vi "NIMS_dfd_Convert Band Specs (Remez Weight).vi"(8 "s":string, 9 "Weight":dbl[](array[numeric]), 10 "A":dbl[](array[numeric]), 11 "F":dbl[](array[numeric])) -> (0 "error out":errorcluster, 1 "freqs of exact gain [Hz]":dbl[](array[numeric]), 2 "band specs":T1[](array[typedef])=[{"band specification"=[{"freq"=0.0, "amplitude"=1.0, "weight"=1.0}, {"freq"=0.2, "amplitude"=1.0, "weight"=1.0}], "ripple constraint"=0.0}, {"band specification"=[{"freq"=0.3, "amplitude"=0.0, "weight"=1.0}, {"freq"=0.5, "amplitude"=0.0, "weight"=1.0}], "ripple constraint"=0.0}])   [LabVIEW 2017, in "NI_DigFilter_MathScript.lvlib"]
uses:
  <vilib>/addons/Digital Filter Design/NI_DigFilter_MathScript.lvlib
  <vilib>/addons/Digital Filter Design/_Objects.llb/DFD Adv Band Spec.ctl
  <vilib>/addons/Digital Filter Design/_Misc.llb/dfd_Error Handlers (Multiple).vi
  <vilib>/addons/Digital Filter Design/NI_DigFilterLicensed.lvlib
panel:
  # "freq"
  # "amplitude"
  # "weight"
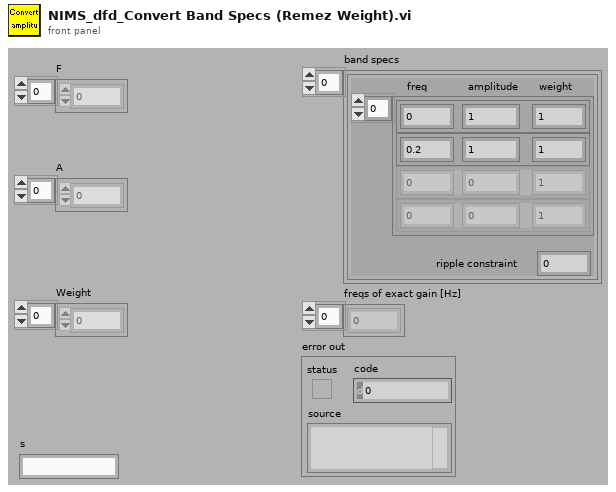
[diagram p1: front panel]
types:
  T1 = typedef "NI_DigFilterLicensed.lvlib/DFD Adv Band Spec.ctl" = cluster{"band specification":cluster{"freq":dbl, "amplitude":dbl, "weight":dbl}[], "ripple constraint":dbl}
  T2 = cluster{cluster{"Numeric":dbl, "Numeric":dbl, "f":dbl}[], dbl}[]
  T3 = cluster{cluster{"Numeric":dbl, "Numeric":dbl, "f":dbl}[], dbl}
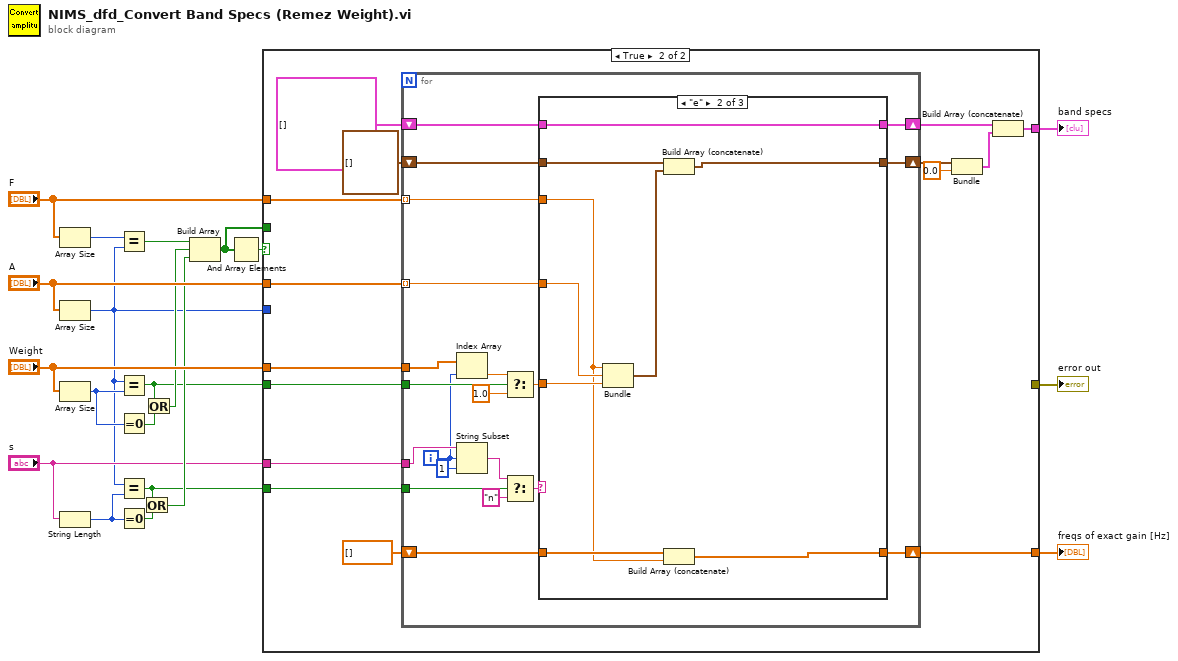
[diagram p0: block diagram]
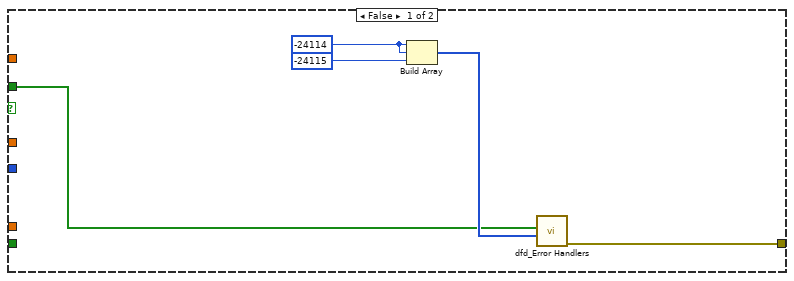
[diagram p2: hidden frame]
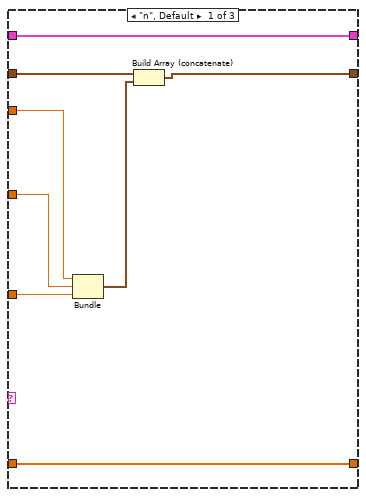
[diagram p3: hidden frame]
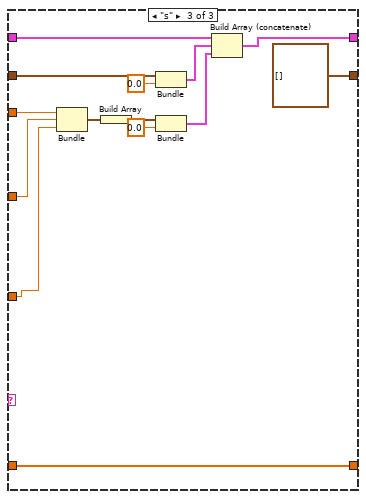
[diagram p4: hidden frame]
diagram:
  n1 = Array Size(array="F") -> (size(s)=w20:i32)
  n2 = Array Size(array="A") -> (size(s)=w6:i32)
  n3 = Array Size(array="Weight") -> (size(s)=w15:i32)
  n4 = String Length(string="s") -> (length=w14:i32)
  n5 = Equal?(x=w20, y=w6) -> (x = y?=w19:bool)
  n6 = Equal?(x=w6, y=w15) -> (x = y?=w8:bool)
  n7 = Equal To 0?(x=w15) -> (x = 0?=w9:bool)
  n8 = Equal?(x=w6, y=w14) -> (x = y?=w7:bool)
  n9 = Equal To 0?(x=w14) -> (x = 0?=w13:bool)
  n10 = Or(x=w7, y=w13) -> (x .or. y?=w11:bool)
  n11 = Or(x=w8, y=w9) -> (x .or. y?=w12:bool)
  n12 = Build Array(w19, w12, w11) -> (w1:bool[])
  n13 = And Array Elements(Boolean array=w1) -> (logical AND=w2:bool)
  n14 = case shown="True" w2 {
    tunnel: "F" -> [_ w40]
    tunnel: "A" -> [_ w39]
    tunnel: "Weight" -> [_ w38]
    tunnel: [w22 _] -> w16
    tunnel: "s" -> [_ w37]
    tunnel: w8 -> [_ w35]
    tunnel: w7 -> [_ w36]
    tunnel: w6 -> [_ _]
    tunnel: [_ w28] -> w4
    tunnel: [_ w27] -> w3
    tunnel: w1 -> [w21 _]
    frame False {
      w23 = -24114 ("element")
      n15 = Build Array(w23, w23, -24115 ("element")) -> (w25:i32[])
      n16 = call-poly <vilib>:"dfd_Error Handlers.vi"("error sources"=w25, "condition failed?"=w21) -> ("error out"=w22:errorcluster)  [unwired: 1 in, 8 out]
    }
    frame True {
      n17 = for {
        tunnel: w40 -> [w50] mode=indexing
        tunnel: w39 -> [w51] mode=indexing
        tunnel: w38 -> [w42]
        tunnel: w37 -> [w60]
        tunnel: w36 -> [w56]
        tunnel: w35 -> [w58]
        shift-right: [w48] -> w31
        shift-left: cluster{"Numeric":dbl, "Numeric":dbl, "f":dbl}[] [] -> [w49]
        shift-right: [w46] -> w27
        shift-left: dbl[] [] -> [w47]
        shift-right: [w44] -> w30
        shift-left: T2 [] -> [w45]
        i -> [w41]
        n18 = Index Array(array=w42, index=w41) -> (element=w43:dbl)
        n19 = String Subset(string=w60, offset (0)=w41, length (rest)=1 ("length (rest)")) -> (substring=w55:string)
        n20 = Select(t=w43, s=w58, f=1.0) -> (s? t:f=w52:dbl)
        n21 = Select(t=w55, s=w56, f="n") -> (s? t:f=w53:string)
        n22 = case shown="\"e\"" w53 {
          tunnel: w52 -> [w66 w76 w87]
          tunnel: w51 -> [w67 w77 w88]
          tunnel: w50 -> [w68 w70 w89]
          tunnel: w49 -> [w65 w75 w91]
          tunnel: [w63 w73 cluster{"Numeric":dbl, "Numeric":dbl, "f":dbl}[] []] -> w48
          tunnel: w47 -> [w62 w72 w78]
          tunnel: [w62 w71 w78] -> w46
          tunnel: w45 -> [w61 w69 w83]
          tunnel: [w61 w69 w80] -> w44
          frame "n", Default {
            n23 = Bundle("Numeric"=w68, "Numeric"=w67, "f"=w66) -> (w64:cluster{"Numeric":dbl, "Numeric":dbl, "f":dbl})  [unwired: 1 out]
            n24 = Build Array (concatenate)(w65, w64) -> (w63:cluster{"Numeric":dbl, "Numeric":dbl, "f":dbl}[])
          }
          frame "e" {
            n25 = Bundle("Numeric"=w70, "Numeric"=w77, "f"=w76) -> (w74:cluster{"Numeric":dbl, "Numeric":dbl, "f":dbl})  [unwired: 1 out]
            n26 = Build Array (concatenate)(w75, w74) -> (w73:cluster{"Numeric":dbl, "Numeric":dbl, "f":dbl}[])
            n27 = Build Array (concatenate)(w72, w70) -> (w71:dbl[])
          }
          frame "s" {
            n28 = Bundle("Numeric"=w89, "Numeric"=w88, "f"=w87) -> (w85:cluster{"Numeric":dbl, "Numeric":dbl, "f":dbl})  [unwired: 1 out]
            n29 = Build Array(w85) -> (w84:cluster{"Numeric":dbl, "Numeric":dbl, "f":dbl}[])
            n30 = Bundle(w91, 0.0) -> (w82:T3)  [unwired: 1 out]
            n31 = Bundle(w84, 0.0) -> (w81:T3)  [unwired: 1 out]
            n32 = Build Array (concatenate)(w83, w82, w81) -> (w80:T2)
          }
        }
      }
      n33 = Bundle(w31, 0.0) -> (w29:T3)  [unwired: 1 out]
      n34 = Build Array (concatenate)(w30, w29) -> (w28:T2)
    }
  }
  "band specs" <- w4
  "error out" <- w16
  "freqs of exact gain [Hz]" <- w3
